vi "S7.vi"(1 "Input array":bool[](array[boolean])) -> (0 "Array":bool[](array[boolean]))   [LabVIEW 2013]
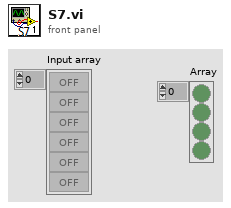
[diagram p1: front panel]
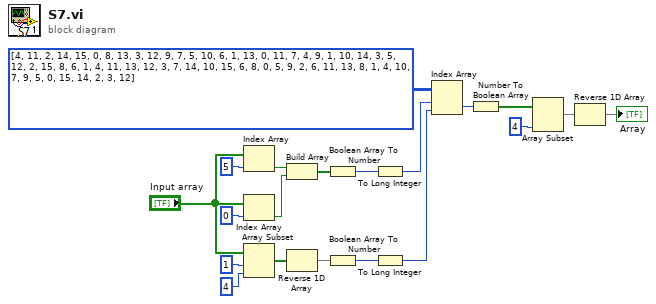
[diagram p0: block diagram]
diagram:
  n1 = Index Array(array="Input array", index=5) -> (element=w4:bool)
  n2 = Index Array(array="Input array", index=0) -> (element=w3:bool)
  n3 = Array Subset(array="Input array", index=1, length=4) -> (w10:bool[])
  n4 = Build Array(w4, w3) -> (w2:bool[])
  n5 = Reverse 1D Array(array=w10) -> (reversed array=w9:bool[])
  n6 = Boolean Array To Number(Boolean array=w2) -> (number=w14:u32)
  n7 = Boolean Array To Number(Boolean array=w9) -> (number=w13:u32)
  n8 = To Long Integer(number=w14) -> (32bit integer=w8:i32)
  n9 = To Long Integer(number=w13) -> (32bit integer=w7:i32)
  n10 = Index Array(array=u8[][] [[4, 11, 2, 14, 15, 0, 8, 13, 3, 12, 9, 7, 5, 10, 6, 1], [13, 0, 11, 7, 4, 9, 1, 10, 14, 3, 5, 12, 2, 15, 8, 6], [1, 4, 11, 13, 12, 3, 7, 14, 10, 15, 6, 8, 0, 5, 9, 2], [6, 11, 13, 8, 1, 4, 10, 7, 9, 5, 0, 15, 14, 2, 3, 12]], index (row)=w8, index (col)=w7) -> (element=w19:u8)
  n11 = Number To Boolean Array(number=w19) -> (Boolean array=w18:bool[])
  n12 = Array Subset(array=w18, length=4) -> (w6:bool[])  [unwired: 1 in]
  n13 = Reverse 1D Array(array=w6) -> (reversed array=→"Array":bool[])
